vi "RT Loop - Watchdog.vi"(8 "FPGA VI Reference Out":refnum<k20>, 11 "Message Queue":refnum<queue>) -> ()   [LabVIEW 2017]
doc: "Send periodic 'pets' to FPGA Main VI to ensure communication is maintained."
uses:
  UI Error Handlers/support/Message Queue/Message Cluster.ctl
  Globals/Global - Configuration Options.vi
  <vilib>/Utility/error.llb/Error Cluster From Error Code.vi
  <vilib>/rvi/errors/niLvFpgaAdjustHostInterfaceError.vi
  Globals/Global - All RT Loop Stop.vi
  <vilib>/rvi/interface/nirviReadWriteControl/nirviReadWriteControl.xnode
  <vilib>/rvi/interface/Simulation/niFpgaSimulationCallBeginRW.vi
  NiFpgaLv.dll
  UI Error Handlers/support/Message Queue/Message Queue.lvlib
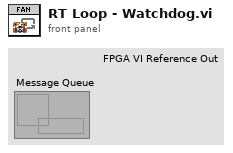
[diagram p1: front panel]
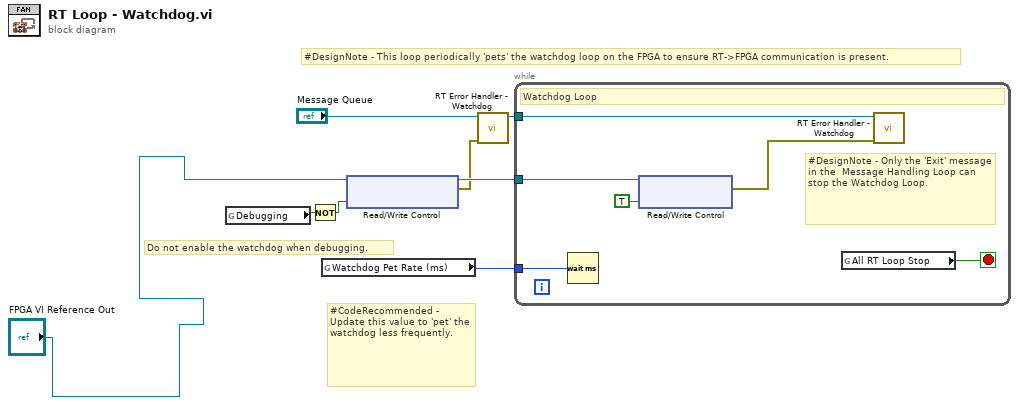
[diagram p0: block diagram]
diagram:
  # "Do not enable the watchdog when debugging."
  # "#CodeRecommended - Update this value to 'pet' the watchdog less frequently."
  # "#DesignNote - This loop periodically 'pets' the watchdog loop on the FPGA to ensure RT->FPGA communication is present."
  n1 = global read "Global - Configuration Options.vi" "Debugging"() -> (w4:bool)
  n2 = Not(x=w4) -> (.not. x?=w3:bool)
  n3 = global read "Global - Configuration Options.vi" "Watchdog Pet Rate (ms)"() -> (w8:u32)
  n4 = xnode "Read/Write Control"("FPGA VI Reference In"="FPGA VI Reference Out", "Enable Watchdog"=w3) -> ("FPGA VI Reference Out"=w7:refnum<k20>, "error out"=w5:errorcluster)  [unwired: 1 in]
  n5 = call "RT Error Handler - Watchdog.vi"("error in (no error)"=w5, "Message Queue"="Message Queue") -> ("dup Message Queue"=w6:refnum<queue>)  [unwired: 9 in]
  n6 = while {
    tunnel: w6 -> [w11]
    tunnel: w7 -> [w14]
    tunnel: w8 -> [w9]
    stop <- w12 stop-if-true
    # "#DesignNote - Only the 'Exit' message in the  Message Handling Loop can stop the Watchdog Loop."
    # "Watchdog Loop"
    n7 = Wait (ms)(milliseconds to wait=w9) -> ()  [unwired: 1 out]
    n8 = xnode "Read/Write Control"("FPGA VI Reference In"=w14, "Pet Watchdog"=TRUE ("Pet RT Watchdog")) -> ("error out"=w10:errorcluster)  [unwired: 1 in, 1 out]
    n9 = global read "Global - All RT Loop Stop.vi" "All RT Loop Stop"() -> (w12:bool)
    n10 = call "RT Error Handler - Watchdog.vi"("error in (no error)"=w10, "Message Queue"=w11) -> ()  [unwired: 9 in, 1 out]
  }
